vi "Sensors Get Values.vi"(1 "Sensors Global Values In":T1) -> (0 "Sensors Global Values Out":T1)   [LabVIEW 2013]
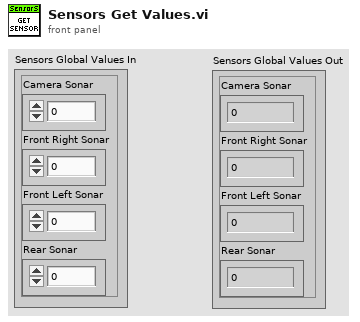
[diagram p1: front panel]
types:
  T1 = cluster{"Camera Sonar":dbl, "Front Right Sonar":dbl, "Front Left Sonar":dbl, "Rear Sonar":dbl}
  T2 = typedef "WPI_AnalogChannelDevRef.ctl" = cluster{"DevStatus":errorcluster, "Analog Module":T3, "Analog Channel":T4}
  T3 = typedef "FPGA_TypedefAnalogModule.ctl" = enum16{"Analog Module 1", "Analog Module 2"}
  T4 = typedef "FPGA_AIChannel.ctl" = enum8{"AI 1", "AI 2", "AI 3", "AI 4", "AI 5", "AI 6", "AI 7", "AI 8", "Invalid"}
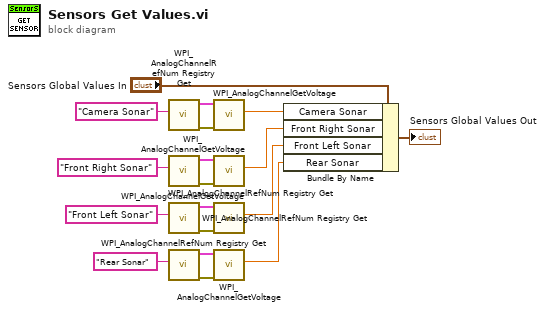
[diagram p0: block diagram]
diagram:
  n1 = call <vilib>:"WPI_AnalogChannelRefNum Registry Get.vi"("refnum name"="Camera Sonar") -> ("error out"=w14:errorcluster, "AIDeviceRef"=w13:T2)  [unwired: 9 in]
  n2 = call <vilib>:"WPI_AnalogChannelRefNum Registry Get.vi"("refnum name"="Front Right Sonar") -> ("error out"=w10:errorcluster, "AIDeviceRef"=w9:T2)  [unwired: 9 in]
  n3 = call <vilib>:"WPI_AnalogChannelRefNum Registry Get.vi"("refnum name"="Front Left Sonar") -> ("error out"=w12:errorcluster, "AIDeviceRef"=w11:T2)  [unwired: 9 in]
  n4 = call <vilib>:"WPI_AnalogChannelRefNum Registry Get.vi"("refnum name"="Rear Sonar") -> ("error out"=w8:errorcluster, "AIDeviceRef"=w7:T2)  [unwired: 9 in]
  n5 = call <vilib>:"WPI_AnalogChannelGetVoltage.vi"("error in (no error)"=w14, "AIDeviceRef"=w13) -> ("Voltage"=w4:dbl)  [unwired: 7 in, 2 out]
  n6 = call <vilib>:"WPI_AnalogChannelGetVoltage.vi"("error in (no error)"=w10, "AIDeviceRef"=w9) -> ("Voltage"=w2:dbl)  [unwired: 7 in, 2 out]
  n7 = call <vilib>:"WPI_AnalogChannelGetVoltage.vi"("error in (no error)"=w12, "AIDeviceRef"=w11) -> ("Voltage"=w3:dbl)  [unwired: 7 in, 2 out]
  n8 = call <vilib>:"WPI_AnalogChannelGetVoltage.vi"("error in (no error)"=w8, "AIDeviceRef"=w7) -> ("Voltage"=w1:dbl)  [unwired: 7 in, 2 out]
  n9 = Bundle By Name(cluster="Sensors Global Values In", "Camera Sonar"=w4, "Front Right Sonar"=w2, "Front Left Sonar"=w3, "Rear Sonar"=w1) -> (→"Sensors Global Values Out":T1)
